vi "Speaker-Play.vi"(6 "Amplitude (V)":dbl=0.1, 7 "Device reference":refnum<vi>, 8 "error in (no error)":errorcluster, 9 "Eventstring":string="auto-generate", 10 "Duration (ms)":dbl=100.0, 11 "Frequency (Hz)":dbl=1000.0) -> (0 "error out":errorcluster)   [LabVIEW 2015]
doc: "Plays a tone (sine wave) on the speaker.\n\nDevice reference: Which speaker?\nFrequency (Hz): Tone frequency\nDuration (ms): Tone duration\nEventstring:\n empty: no timestamp\n unwired or \"auto-generate\":\n [name].play:[freq]Hz,[duration]ms\n otherwise: timestamp w/ provided string\n\nIf you try to play more than one tone at a time, they will just get queued."
uses:
  Typedefs/Speaker.ctl
  Rack/Typedefs/OutputRequest refnum.ctl
  Rack/Typedefs/OutputRequest.ctl
  Rack/Typedefs/InputData cluster.ctl
  Rack/Methods/Port drivers/DigitalInput-DataCluster.ctl
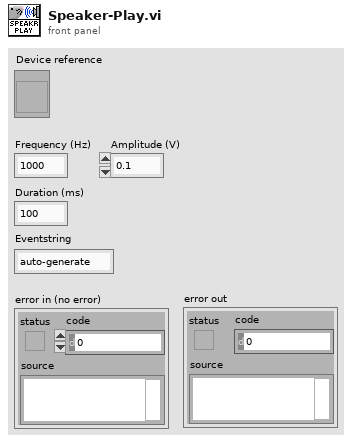
[diagram p1: front panel]
types:
  T1 = cluster{"Waveform type":enum16{"sine"}, "Amplitude (V)":dbl, "Sample clock (Hz)":dbl}
  T2 = typedef "Speaker.ctl" = cluster{"Settings":cluster{"Portname":string, "Index":i32, "Timestamp portname":string}, "OutputRequest event ref":T3, "InputData reference":refnum<vi>}
  T3 = typedef "OutputRequest refnum.ctl" = refnum<user-event>
  T4 = typedef "OutputRequest.ctl" = cluster{"Target":string, "Command":string}
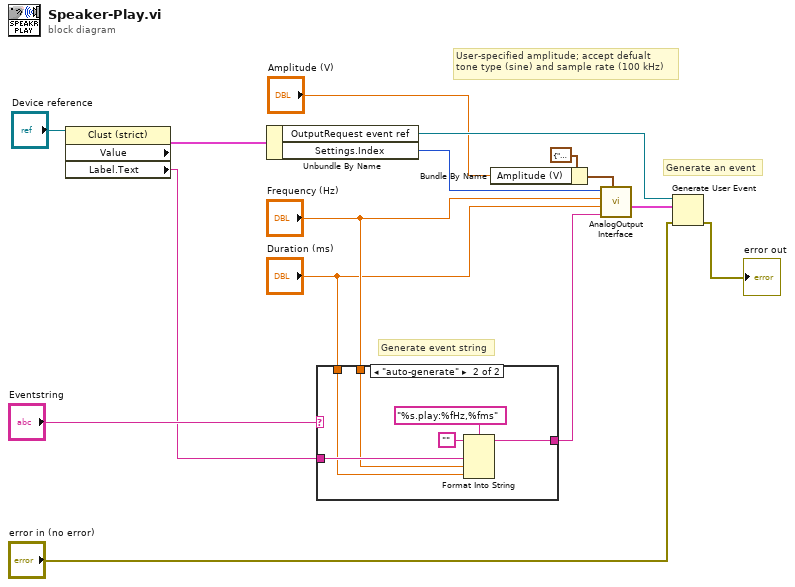
[diagram p0: block diagram]
diagram:
  # "User-specified amplitude; accept defualt\ntone type (sine) and sample rate (100 kHz)"
  # "Generate event string"
  # "Generate an event"
  n1 = property class="Clust (strict)"(reference="Device reference") -> ("Value"=w14:T2, "Label.Text"=w6:string)  [unwired: 1 in, 2 out]
  n2 = Unbundle By Name(w14) -> ("OutputRequest event ref"=w12:T3, "Settings.Index"=w8:i32)
  n3 = case shown="\"auto-generate\"" "Eventstring" {
    selector: "Eventstring" -> [w16 _]
    tunnel: w6 -> [_ w20]
    tunnel: [w16 w19] -> w3
    tunnel: "Frequency (Hz)" -> [_ w18]
    tunnel: "Duration (ms)" -> [_ w17]
    frame Default {
      # "Use user-provided string"
    }
    frame "auto-generate" {
      n4 = Format Into String(format string="%s.play:%fHz,%fms", initial string="", w20, w18, w17) -> (resulting string=w19:string)  [unwired: 1 in, 1 out]
    }
  }
  n5 = Bundle By Name(cluster=T1 {"Waveform type"=enum."sine", "Amplitude (V)"=1.0, "Sample clock (Hz)"=100000.0} ("Options"), "Amplitude (V)"="Amplitude (V)") -> (w11:T1)
  n6 = call "AnalogOutput Interface.vi"("Options"=w11, "Eventstring"=w3, "Duration (ms)"="Duration (ms)", "Frequency (Hz)"="Frequency (Hz)", "Port index"=w8) -> ("OutputRequest"=w13:T4)  [unwired: 6 in]
  n7 = Generate User Event(user event=w12, event data cluster=w13, error in="error in (no error)") -> (error out=→"error out":errorcluster)  [unwired: 1 in, 1 out]
